vi "Camera.IMAQdx.Connect_LL.vi"(8 "Error In":errorcluster, 11 "Interface":string) -> (0 "Error Out":errorcluster, 3 "Session Out":T1)   [LabVIEW 2017, in "Camera_IMAQdx.lvclass"]
uses:
  Camera_IMAQdx.lvclass
  <vilib>/userdefined/High Color/IMAQdx.ctl
  <vilib>/vision/driver/IMAQdx.llb/IMAQdx Camera Control Mode.ctl
  <vilib>/vision/driver/NI_Vision_Acquisition_Software.lvlib
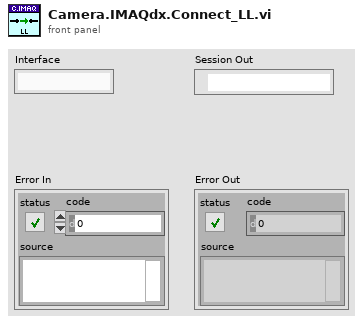
[diagram p1: front panel]
types:
  T1 = typedef "IMAQdx.ctl" = refnum<k21>
  T2 = typedef "NI_Vision_Acquisition_Software.lvlib/IMAQdx Camera Control Mode.ctl" = enum32{"Controller", "Listener"}
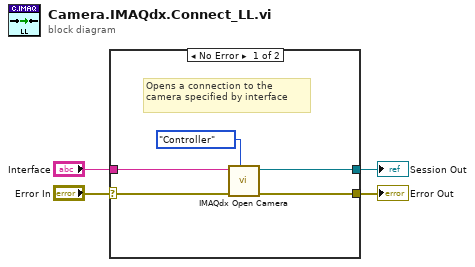
[diagram p0: block diagram]
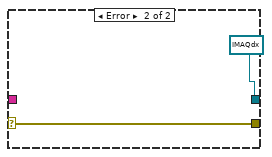
[diagram p2: hidden frame]
diagram:
  n1 = case shown="No Error" "Error In" {
    selector: "Error In" -> [w9 w11]
    tunnel: [w7 w11] -> w3
    tunnel: "Interface" -> [w8 _]
    tunnel: [w5 T1 refnum ("Session Out")] -> w1
    frame No Error {
      # "Opens a connection to the camera specified by interface"
      n2 = call <vilib>:"IMAQdx Open Camera.vi"("Camera Control Mode"=IMAQdx_Camera_Control_Mode."Controller", "error in"=w9, "Session In"=w8) -> ("error out"=w7:errorcluster, "Session Out"=w5:T1)  [unwired: 7 out]
    }
    frame Error {
    }
  }
  "Error Out" <- w3
  "Session Out" <- w1
